vi "Stop Core.vi"(10 "final error code":i32, 11 "Sounds in":refnum<class "Sounds.lvclass">) -> (3 "Sounds out":refnum<class "Sounds.lvclass">)   [LabVIEW 2024, in "Sounds.lvlib" / "Sounds.lvclass"]
doc: "<p>(<strong>Filename</strong>: <span class=\"dnl\">Actor Framework.lvlib:Actor.lvclass:Stop Core.vi</span>)</p>\n<p>Defines what the actor does before it stops. Use the <strong>final error code</strong> input to determine whether the actor shut down in response to an error.</p>\n<p>By default, this method passes the Stop message along to all <a href=\"nihelplauncher://docs/csh?context=lvcore_lvcomm_af_launch_nested_actor\">auto-stop nested actors</a>. A descendant class may override this method to define additional behavior, such as shutting down any processes the actor initiated in its override of the <a href=\"nihelplauncher://docs/csh?context=lvcore_lvcomm_af_actor_core\">Actor Core</a> method.</p>"
uses:
  Sounds.lvclass
  Sounds.lvclass/Sounds.ctl
  <vilib>/ActorFramework/Actor/Actor.lvclass
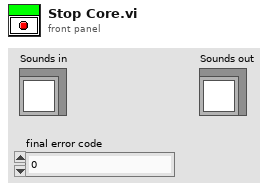
[diagram p1: front panel]
types:
  T1 = typedef "Sound Output Task ID.ctl" = u32
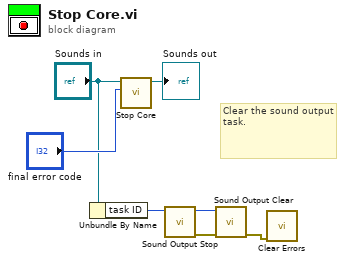
[diagram p0: block diagram]
diagram:
  # "Clear the sound output task."
  n1 = Unbundle By Name("Sounds in") -> ("task ID"=w4:T1)
  n2 = call-parent "Stop Core.vi"("final error code"="final error code", "Actor in"="Sounds in") -> ("Actor out"=→"Sounds out":refnum<class "Sounds.lvclass">)  [unwired: 9 in]
  n3 = call <vilib>:"Sound Output Stop.vi"("task ID"=w4) -> ("error out"=w2:errorcluster, "task ID out"=w3:T1)  [unwired: 9 in]
  n4 = call <vilib>:"Sound Output Clear.vi"("error in (no error)"=w2, "task ID"=w3) -> ("error out"=w1:errorcluster)  [unwired: 9 in]
  n5 = call <vilib>:"Clear Errors.vi"("error in (no error)"=w1) -> ()  [unwired: 5 in, 2 out]
